vi "Parse updateChatLastMessage.vi"(8 "error in (no error)":errorcluster, 11 "JSON (UTF-8) String":string) -> (0 "error out":errorcluster, 2 "Telegram State":T1, 3 "Variant":variant)   [LabVIEW 2015, in "JSON Library.lvlib"]
doc: "Created IvanLis by LabVIEW Portal\nProfile: http://labviewportal.org/memberlist.php?mode=viewprofile&u=987\neMail: IvanLisanov@gMail.com\nTelegram: https://t.me/IvanLis"
uses:
  JSON Library.lvlib
  Telegram Library/TypeDef/Telegram State.ctl
  TypeDef/Message Text.ctl
  Telegram Library/Telegram Library.lvlib
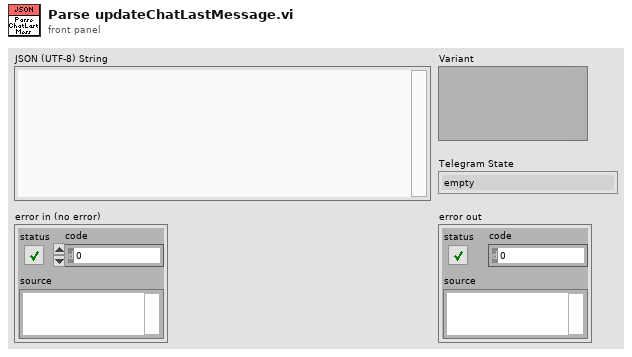
[diagram p1: front panel]
types:
  T1 = typedef "Telegram Library.lvlib/Telegram State.ctl" = enum16{"empty", "ok", "authorizationStateClosed", "authorizationStateWaitTdlibParameters", "authorizationStateWaitEncryptionKey", "authorizationStateWaitPhoneNumber", "authorizationStateWaitCode", "connectionStateWaitingForNetwork", "connectionStateConnectingToProxy", "connectionStateUpdating", "connectionStateConnecting", "connectionStateReady", "updateUser_user", "updateNewChat_chat", "updateNewMessage_Text", "updateChatLastMessage_Text", "updateDeleteMessages", "updateChatPosition", "ChatHistoryMessages_Text"}
  T2 = typedef "JSON Library.lvlib/Message Text.ctl" = cluster{"@type":string, "id":i64, "sender_id":cluster{"@type":string, "user_id":i64}, "chat_id":i64, "date":i64, "content":cluster{"@type":string, "text":cluster{"@type":string, "text":string}}}
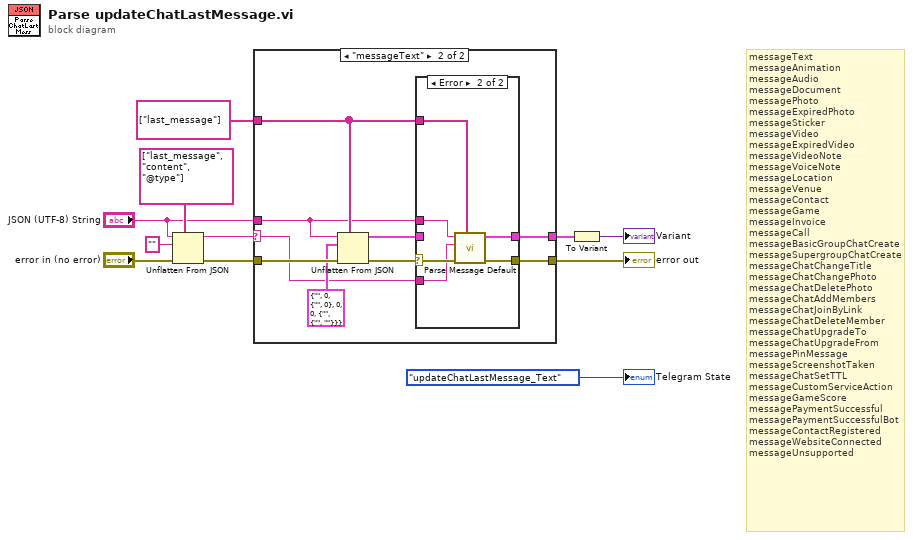
[diagram p0: block diagram]
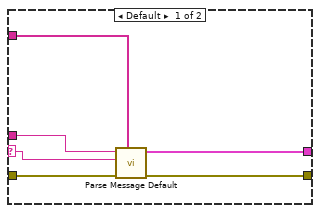
[diagram p2: hidden frame]
diagram:
  # "messageText\nmessageAnimation\nmessageAudio\nmessageDocument\nmessagePhoto\nmessageExpiredPhoto\nmessageSticker\nmessageVideo\nmessageExpiredVideo\nmessageVideoNote\nmessageVoiceNote\nmessageLocation\nmessageVenue\nmessageContact\nmessageGame\nmessageInvoice\nmessageCall\nmessageBasicGroupChatCreate\nmessageSupergroupChatCreate\nmessageChatChangeTitle\nmessageChatChangePhoto\nmessageChatDeletePhoto\nmessageChatAddMembers\nmessageChatJoinByLink\nmessageChatDeleteMember\nmessageChatUpgradeTo\nmessageChatUpgradeFrom\nmessagePinMessage\nmessageScreenshotTaken\nmessageChatSetTTL\nmessageCustomServiceAction\nmessageGameScore\nmessagePaymentSuccessful\nmessagePaymentSuccessfulBot\nmessageContactRegistered\nmessageWebsiteConnected\nmessageUnsupported"
  n1 = Unflatten From JSON(path=string[] ["last_message", "content", "@type"], JSON string="JSON (UTF-8) String", type and defaults="", error in (no error)="error in (no error)") -> (value=w10:string, error out=w7:errorcluster)  [unwired: 3 in]
  n2 = case shown="\"messageText\"" w10 {
    selector: w10 -> [w13 w18]
    tunnel: w7 -> [w17 w26]
    tunnel: [w16 w23] -> w3
    tunnel: "JSON (UTF-8) String" -> [w14 w19]
    tunnel: [w12 w21] -> w8
    tunnel: string[] ["last_message"] ("path") -> [w15 w20]
    frame Default {
      n3 = call "Parse Message Default.vi"("path"=w15, "error in (no error)"=w17, "content.@type"=w13, "JSON (UTF-8) String"=w14) -> ("error out"=w16:errorcluster, "New Message Text"=w12:T2)  [unwired: 6 in]
    }
    frame "messageText" {
      n4 = Unflatten From JSON(path=w20, JSON string=w19, type and defaults=T2 {"@type"="", "id"=0, "sender_id"={"@type"="", "user_id"=0}, "chat_id"=0, "date"=0, "content"={"@type"="", "text"={"@type"="", "text"=""}}} ("Message Text"), error in (no error)=w26) -> (value=w22:T2, error out=w24:errorcluster)  [unwired: 3 in]
      n5 = case shown="Error" w24 {
        selector: w24 -> [w28 w34]
        tunnel: [w28 w33] -> w23
        tunnel: w22 -> [w27 _]
        tunnel: [w27 w29] -> w21
        tunnel: w20 -> [_ w32]
        tunnel: w19 -> [_ w31]
        tunnel: w18 -> [_ w30]
        frame No Error {
        }
        frame Error {
          n6 = call "Parse Message Default.vi"("path"=w32, "error in (no error)"=w34, "content.@type"=w30, "JSON (UTF-8) String"=w31) -> ("error out"=w33:errorcluster, "New Message Text"=w29:T2)  [unwired: 6 in]
        }
      }
    }
  }
  "error out" <- w3
  n7 = To Variant(anything=w8) -> (Variant=→"Variant":variant)
  "Telegram State" <- Telegram_State."updateChatLastMessage_Text" ("Telegram State")
